vi "Configure Channels.vi"(8 "error in (no error)":errorcluster, 11 "Scope Base CFG in":refnum<class "Scope Base CFG.lvclass">) -> (0 "error out":errorcluster, 3 "Scope Base CFG out":refnum<class "Scope Base CFG.lvclass">)   [LabVIEW 2023, in "Scope Base CFG.lvclass"]
uses:
  Scope Base CFG.lvclass
  Scope Base CFG.lvclass/Scope Base CFG.ctl
  <vilib>/ErrorRing/Error Ring.xnode
  <vilib>/Utility/error.llb/Error Cluster From Error Code.vi
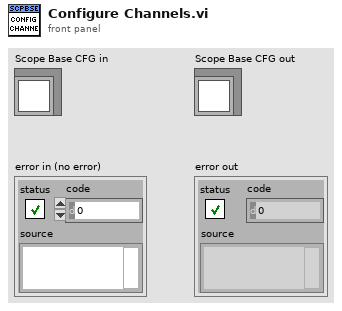
[diagram p1: front panel]
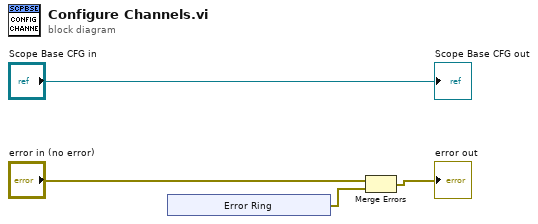
[diagram p0: block diagram]
diagram:
  n1 = xnode "Error Ring"() -> ("error out"=w1:errorcluster)
  n2 = Merge Errors("error in (no error)", w1) -> (→"error out":errorcluster)
  "Scope Base CFG out" <- "Scope Base CFG in"
